vi "write_tdms_file.vi"(8 "error in (no error)":errorcluster caption="错误输入（无错误）", 10 "waveform array":waveform(sgl)[](array[waveform]) caption="波形数组", 11 "tdms file ref in":refnum<k34> caption="TDMS文件引用输入") -> (0 "error out":errorcluster caption="错误输出", 3 "tdms file ref out":refnum<k34> caption="TDMS文件引用输出")   [LabVIEW 2015]
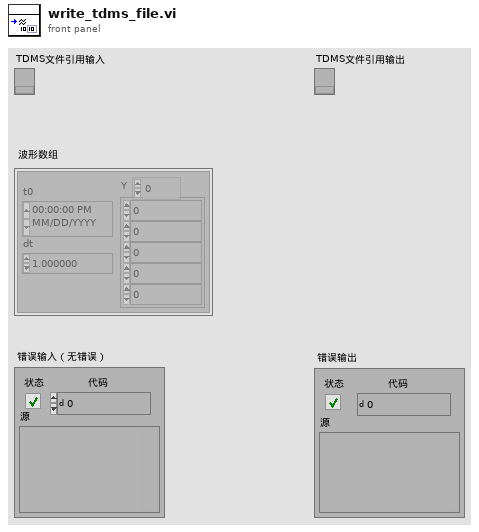
[diagram p1: front panel]
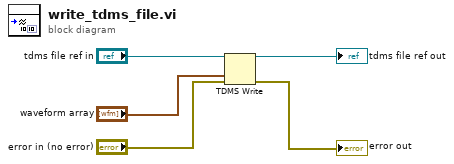
[diagram p0: block diagram]
diagram:
  n1 = TDMS Write(0:"tdms file ref in", 9:"waveform array", 11:"error in (no error)") -> (4:→"tdms file ref out":refnum<k34>, 15:→"error out":errorcluster)  [unwired: 3 in, 2 out]
